vi "OneDigitTo2DigitWith0.vi"(10 "number":i32) -> (2 "output":string)   [LabVIEW 2012]
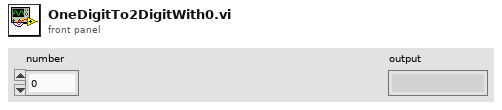
[diagram p1: front panel]
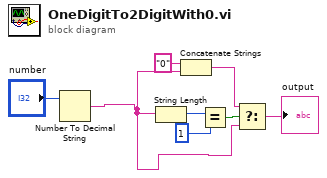
[diagram p0: block diagram]
diagram:
  n1 = Number To Decimal String(number="number") -> (decimal integer string=w2:string)  [unwired: 1 in]
  n2 = String Length(string=w2) -> (length=w8:i32)
  n3 = Concatenate Strings("0" ("string"), w2) -> (w4:string)
  n4 = Equal?(x=w8, y=1) -> (x = y?=w6:bool)
  n5 = Select(t=w4, s=w6, f=w2) -> (s? t:f=→"output":string)
